vi "Read TEC_AO.vi"(8 "error in (no error)":errorcluster, 11 "TEC Humidity Control in":refnum<class "TEC Humidity Control.lvclass">) -> (0 "error out":errorcluster, 2 "TEC_AO":refnum<k21>, 3 "TEC Humidity Control out":refnum<class "TEC Humidity Control.lvclass">)   [LabVIEW 2016, in "TEC Humidity Control.lvclass"]
uses:
  TEC Humidity Control.lvclass
  TEC Humidity Control.lvclass/TEC Humidity Control.ctl
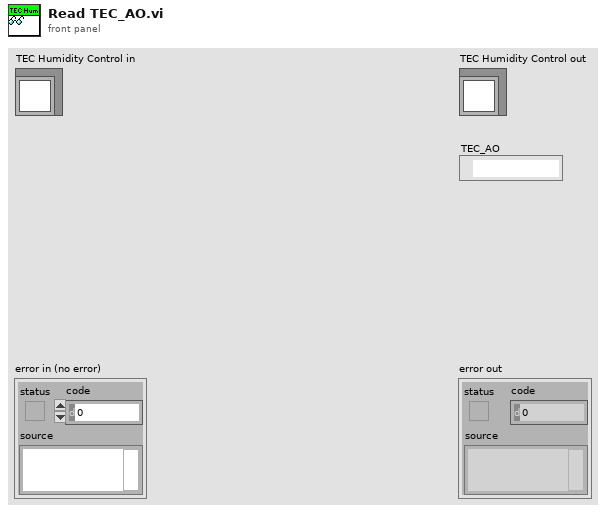
[diagram p1: front panel]
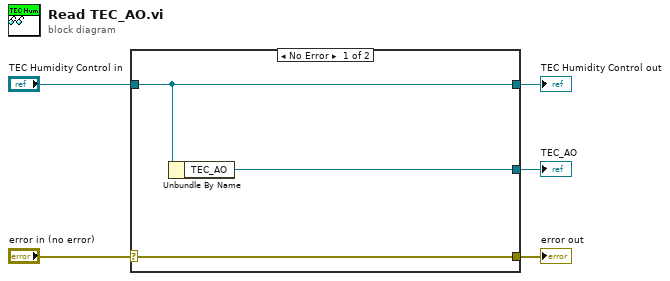
[diagram p0: block diagram]
diagram:
  n1 = case shown="No Error" "error in (no error)" {
    selector: "error in (no error)" -> [w8 w9]
    tunnel: [w8 w9] -> w4
    tunnel: [w7 w10] -> w2
    tunnel: "TEC Humidity Control in" -> [w7 w10]
    tunnel: [w6 _] -> w1
    frame No Error {
      n2 = Unbundle By Name(w7) -> ("TEC_AO"=w6:refnum<k21>)
    }
    frame Error {
    }
  }
  "error out" <- w4
  "TEC Humidity Control out" <- w2
  "TEC_AO" <- w1
